vi "Ex1 (vetori si matrici).vi"() -> ()   [LabVIEW 2023]
panel:
  out "Numar valori":dbl
  in  "Array":dbl[](array[numeric])
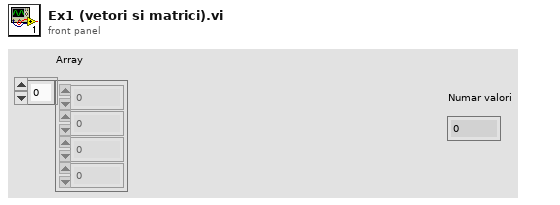
[diagram p1: front panel]
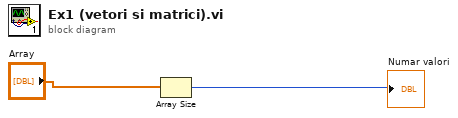
[diagram p0: block diagram]
diagram:
  n1 = Array Size(array="Array") -> (size(s)=→"Numar valori":i32)
